vi "Loop Tunnel Modes.vi"() -> ()   [LabVIEW 2023]
doc: "Takes a 2D array, a maximum and a minimum, and returns an array of out of range elements. This example demonstrates the use of conditional auto-indexing loop tunnels and auto-concatenating loop tunnels."
panel:
  in  "Bad Range Message":string="Minimum is not less than Maximum"
  out "Number of Elements Out of Range":i32
  out "Out of Range Elements":dbl[](array[numeric])
  in  "Minimum":dbl=2.0
  in  "Maximum":dbl=5.0
  in  "Input Array":dbl[][](array[numeric])=[[5.0, 3.0, 1.0], [10.0, 59.0, 12.0], [33.0, 2.0, 39.0], [91.0, 7.0, 10.0], [7.0, 8.0, 25.0]]
  # "Overview: Demonstrates the use of Conditional Loop Tunnels and Concatenating Loop Tunnels.\nInstructions:\n1. Run the VI. Verify that all of the Out of Range Elements are outside the specified Minimum and Maximum values.\n2. Change the Minimum and Maximum values and run the VI again."
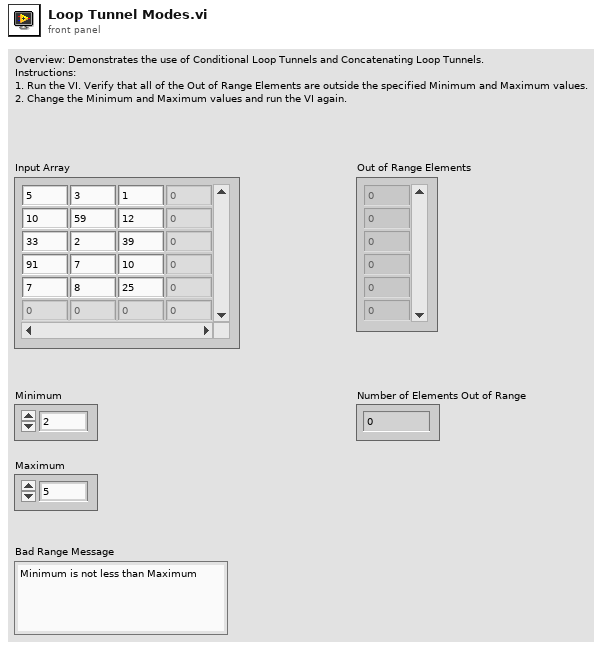
[diagram p1: front panel]
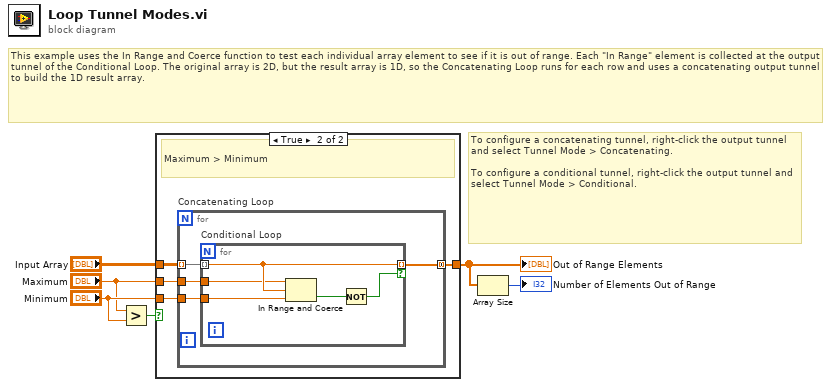
[diagram p0: block diagram]
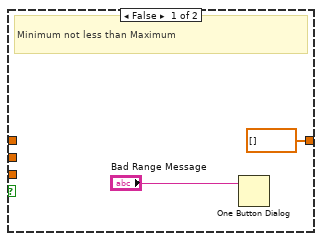
[diagram p2: hidden frame]
diagram:
  # "To configure a concatenating tunnel, right-click the output tunnel and select Tunnel Mode > Concatenating.\n\nTo configure a conditional tunnel, right-click the output tunnel and select Tunnel Mode > Conditional."
  # "This example uses the In Range and Coerce function to test each individual array element to see if it is out of range. Each \"In Range\" element is collected at the output tunnel of the Conditional Loop. The original array is 2D, but the result array is 1D, so the Concatenating Loop runs for each row and uses a concatenating output tunnel to build the 1D result array."
  n1 = Greater?(x="Maximum", y="Minimum") -> (0:w3:bool)
  n2 = case shown="True" w3 {
    tunnel: "Input Array" -> [_ w12]
    tunnel: "Maximum" -> [_ w11]
    tunnel: "Minimum" -> [_ w10]
    tunnel: [dbl[] [] w9] -> w2
    frame False {
      # "Minimum not less than Maximum"
      n3 = One Button Dialog(message="Bad Range Message") -> ()  [unwired: 1 in, 1 out]
    }
    frame True {
      # "Maximum > Minimum"
      n4 = for "Concatenating Loop" {
        tunnel: w12 -> [w16] mode=indexing
        tunnel: w11 -> [w15]
        tunnel: w10 -> [w14]
        tunnel: [w13] -> w9 mode=concatenating
        n5 = for "Conditional Loop" {
          tunnel: w16 -> [w21] mode=indexing
          tunnel: w15 -> [w20]
          tunnel: w14 -> [w19]
          tunnel: [w21] -> w13 mode=indexing if=w17
          n6 = In Range and Coerce(upper limit=w20, x=w21, lower limit=w19) -> (In Range?=w18:bool)  [unwired: 1 out]
          n7 = Not(x=w18) -> (.not. x?=w17:bool)
        }
      }
    }
  }
  "Out of Range Elements" <- w2
  n8 = Array Size(array=w2) -> (size(s)=→"Number of Elements Out of Range":i32)
